vi "Direct.vi"(7 "Actor in":refnum<class "Actor.lvclass">) -> (0 "Error out":errorcluster, 5 "Actor out":refnum<class "Actor.lvclass">)   [LabVIEW 2025, in "jettl.lvlib" / "Destroy Msg.lvlib"]
uses:
  Destroy Msg.lvlib
  Actor/Actor/Actor.lvclass
  Destroy Msg/Destroy Msg.lvclass
  Actor/Actor.lvlib
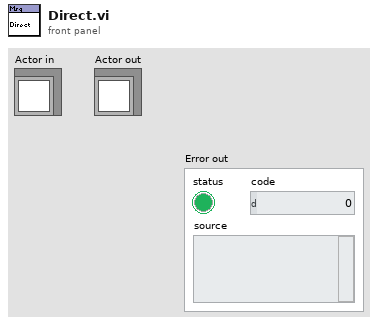
[diagram p1: front panel]
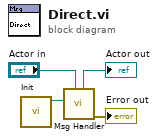
[diagram p0: block diagram]
diagram:
  n1 = call "Init.vi"() -> ("Destroy Msg out"=w1:refnum<class "Destroy Msg.lvclass">)  [unwired: 11 in]
  n2 = call "Msg Handler.vi"("Actor in"="Actor in", "Msg"=w1) -> ("Error out"=→"Error out":errorcluster, "Actor out"=→"Actor out":refnum<class "Actor.lvclass">)  [unwired: 8 in]
